vi "设置颜色.vi"(8 "错误输入（无错误）":errorcluster, 11 "XY图输入":refnum<vi>) -> (0 "错误输出":errorcluster)   [LabVIEW 2021]
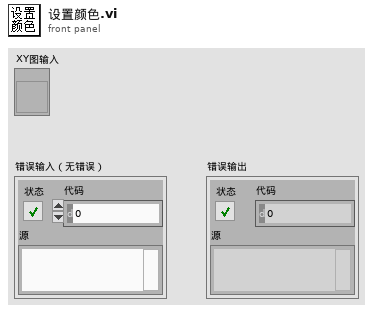
[diagram p1: front panel]
types:
  T1 = typedef "曲线属性.ctl" = cluster{"曲线名":string, "曲线颜色":u32}
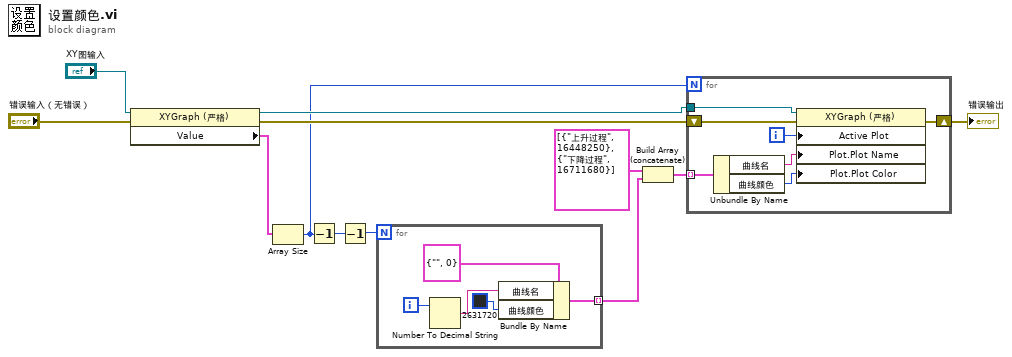
[diagram p0: block diagram]
diagram:
  n1 = property on="属性节点" class="XYGraph (严格)"(reference="XY图输入", error in="错误输入（无错误）") -> (reference out=w2:refnum<vi>, error out=w11:errorcluster, "Value"=w8:cluster{"测试数据":dbl[], "测试数据":dbl[]}[])
  n2 = Array Size(array=w8) -> (size(s)=w1:i32)
  n3 = Decrement(x=w1) -> (x-1=w10:i32)
  n4 = Decrement(x=w10) -> (x-1=w9:i32)
  n5 = for {
    N: w9 -> [_]
    tunnel: [w13] -> w5 mode=indexing
    i -> [w14]
    n6 = Number To Decimal String(number=w14) -> (decimal integer string=w15:string)  [unwired: 1 in]
    n7 = Bundle By Name(cluster=T1 {"曲线名"="", "曲线颜色"=0} ("曲线属性"), "曲线名"=w15, "曲线颜色"=u32 2631720) -> (w13:T1)
  }
  n8 = Build Array (concatenate)(T1[] [{"曲线名"="上升过程", "曲线颜色"=16448250}, {"曲线名"="下降过程", "曲线颜色"=16711680}], w5) -> (w7:T1[])
  n9 = for {
    N: w1 -> [_]
    tunnel: w7 -> [w22] mode=indexing
    shift-right: [w19] -> w12
    shift-left: w11 -> [w20]
    tunnel: w2 -> [w18]
    i -> [w24]
    n10 = Unbundle By Name(w22) -> ("曲线名"=w23:string, "曲线颜色"=w21:u32)
    n11 = property on="属性节点" class="XYGraph (严格)"(reference=w18, error in=w20, "Active Plot"=w24, "Plot.Plot Name"=w23, "Plot.Plot Color"=w21) -> (error out=w19:errorcluster)  [unwired: 1 out]
  }
  "错误输出" <- w12
